vi "Fast Get Item Property (Dependent Node Pointer) FuncGlobal.vi"(5 "Action":enum16{"Open or Add", "Close Ref"}(ring), 8 "error in (no error)":errorcluster, 10 "Property Name":string, 11 "Item Ref in":T1 format="%.0x") -> (0 "error out":errorcluster, 1 "Dependent Node Ref":T1=18446744073709551615 format="%.0x", 3 "Item Ref out":T1 format="%.0x", 4 "Found":bool)   [LabVIEW 2011]
doc: "Returns the <B>Value</B> of a specific item <B>Property Name</B>. If the <B>Property Name</B> does not exist for the specified item, <B>Value</B> returns <B>Default Value</B>."
uses:
  <vilib>/NI Veristand/Custom Device API/Custom Device Item Ref.ctl
  <vilib>/NI Veristand/Custom Device API/Custom Device API.lvlib
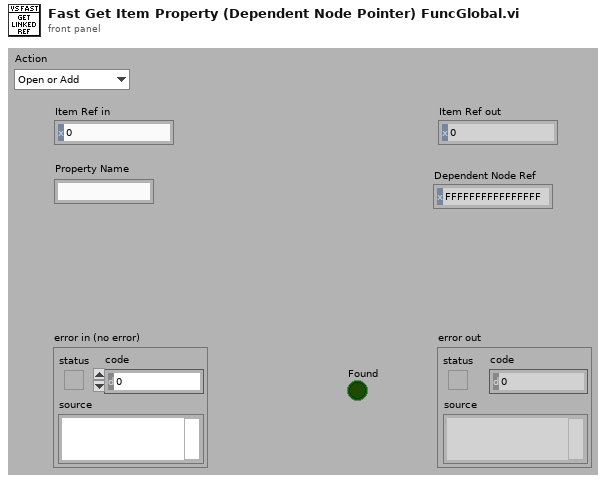
[diagram p1: front panel]
types:
  T1 = typedef "Custom Device API.lvlib/Custom Device Item Ref.ctl" = u64
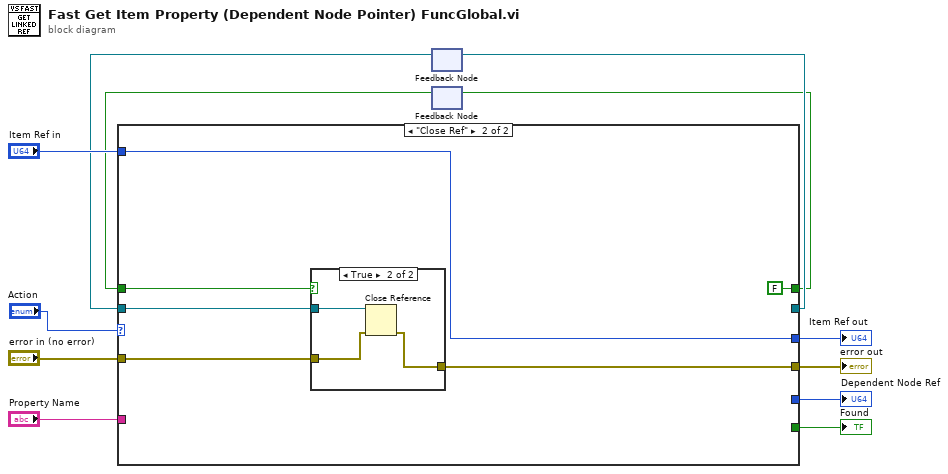
[diagram p0: block diagram]
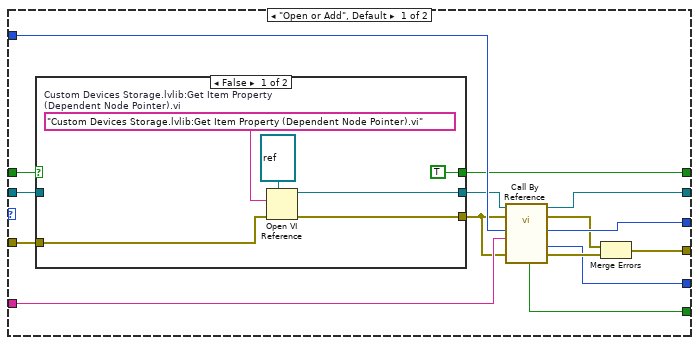
[diagram p2: hidden frame]
diagram:
  n1 = feedback #1() -> (w2:refnum<vi>)  [unwired: 1 in]
  n2 = feedback #2() -> (w3:bool)  [unwired: 1 in]
  n3 = case shown="\"Close Ref\"" "Action" {
    tunnel: [w26 _] -> w5
    tunnel: "error in (no error)" -> [w25 w41]
    tunnel: "Item Ref in" -> [w24 w39]
    tunnel: [w23 w39] -> w10
    tunnel: [w22 w38] -> w9
    tunnel: "Property Name" -> [w21 _]
    tunnel: [w20 _] -> w7
    tunnel: [w19 _] -> w6
    tunnel: [w15 FALSE] -> w4
    tunnel: w3 -> [w14 w37]
    tunnel: w2 -> [w13 w42]
    frame "Open or Add", Default {
      n4 = case shown="False" w14 {
        selector: w14 -> [_ w36]
        tunnel: w25 -> [w31 w34]
        tunnel: [w30 w35] -> w18
        tunnel: [w29 w34] -> w17
        tunnel: [TRUE w36] -> w15
        tunnel: w13 -> [_ w35]
        frame False {
          w33 = "Custom Devices Storage.lvlib:Get Item Property (Dependent Node Pointer).vi"  # Custom Devices Storage.lvlib:Get Item Property (Dependent Node Pointer).vi
          n5 = Open VI Reference(type specifier VI Refnum (for type only)=refnum<vi> refnum, vi path=w33, error in (no error)=w31) -> (vi reference=w30:refnum<vi>, error out=w29:errorcluster)  [unwired: 3 out]
        }
        frame True {
        }
      }
      n6 = call-by-ref "?"(reference=w18, error in=w17, 8:"error in (no error)"=w17, "Property Name"=w21, "Item Ref in"=w24) -> (reference out=w26:refnum<vi>, error out=w16:errorcluster, 0:"error out"=w27:errorcluster, "Dependent Node"=w19:T1, "Item Ref out"=w23:T1, "Found?"=w20:bool)  [unwired: 5 in]
      n7 = Merge Errors(w16, w27) -> (w22:errorcluster)
    }
    frame "Close Ref" {
      n8 = case shown="True" w37 {
        tunnel: w42 -> [_ w46]
        tunnel: w41 -> [w43 w45]
        tunnel: [w43 w44] -> w38
        frame False {
        }
        frame True {
          n9 = Close Reference(reference=w46, error in (no error)=w45) -> (error out=w44:errorcluster)
        }
      }
    }
  }
  "Item Ref out" <- w10
  "error out" <- w9
  "Found" <- w7
  "Dependent Node Ref" <- w6
  n10 = feedback-in #1(w5) -> ()
  n11 = feedback-in #2(w4) -> ()
